vi "Generate All Combinations of N-Dimensional Coordinates Ver05.vi"(4 "Delete ROWS w/\nCOL #2 > #1":bool, 5 "Delete ROWS w/\nCOL #1 > #0":bool, 6 "INDEX of \nCOLS to Use":dbl[](array[numeric])=[0.0, 1.0, 2.0], 7 "Delete ROWS w/\nCOL #2 < #0":bool, 8 "Delete ROW if\nContains #":dbl=99.99, 10 "2D Big Data Array":dbl[][](array[numeric])=[[66.0, 11.0, 111.0], [2.0, 22.0, 9.0]]) -> (3 "FINAL ARRAY":dbl[][](array[numeric]))   [LabVIEW 2017]
uses:
  <vilib>/Analysis/Matrix/Numeric/Conversions/Array To Matrix - RA2.vi
  <vilib>/Analysis/Matrix/Numeric/Conversions/Matrix To Array - RM.vi
  <vilib>/Analysis/Matrix/NI_Matrix.lvlib
panel:
  in  "Tab Control":T1(tab)
  out "All COMBINATIONS of Numbers in Selected COLS":dbl[][](array[numeric])
  out "1st Condition Applied (Remove \nColumns with COL#1 > COL#0)":dbl[][](array[numeric])
  out "2nd Condition Applied (Remove \nColumns with COL#2 > COL#1)":dbl[][](array[numeric])
  out "FINAL # of ROWS":i32
  out "Selected COLS":dbl[][](array[numeric])
  out "# Dimensions \nSelected":i32
  # "COL#0"
  # "COL#1"
  # "COL#2"
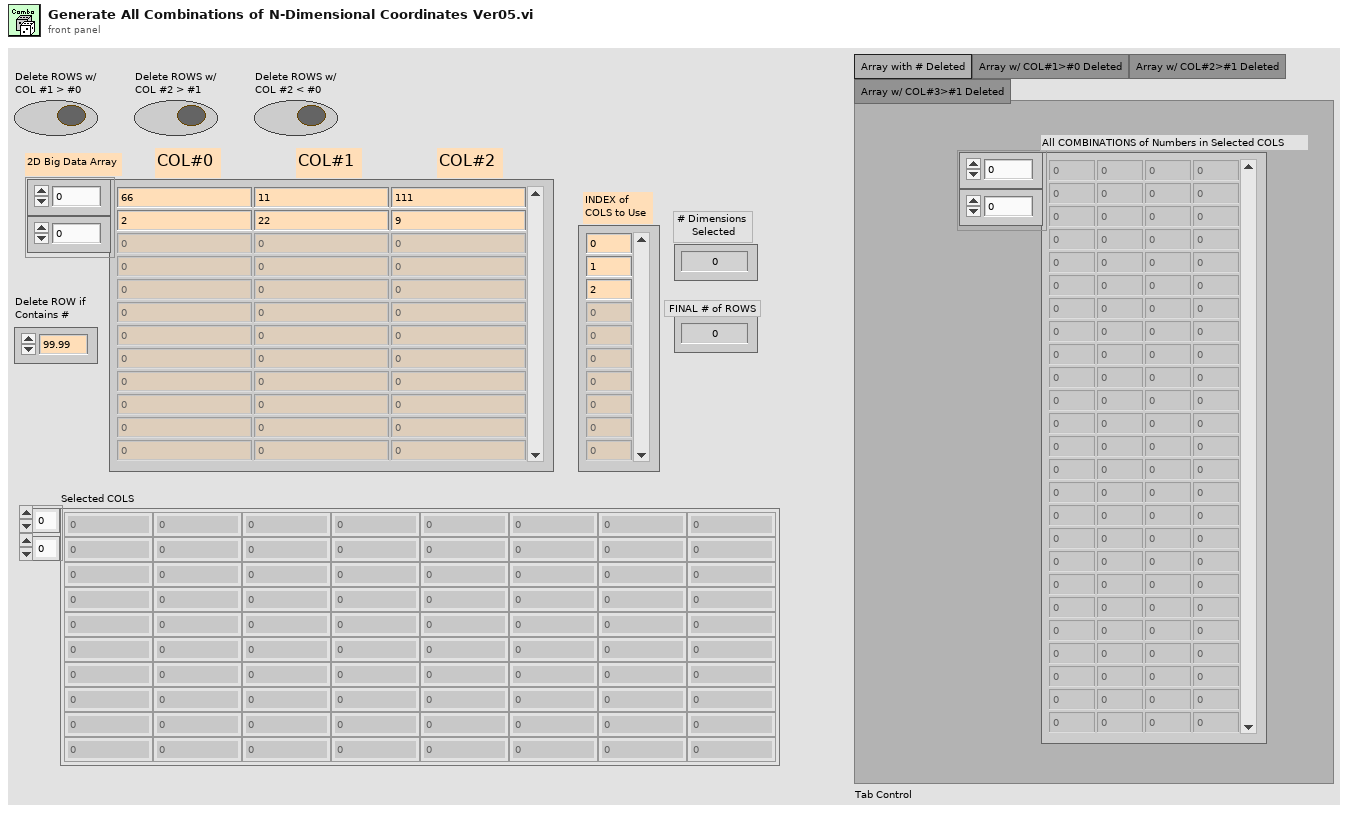
[diagram p1: front panel]
types:
  T1 = enum32{"Array with # Deleted", "Array w/ COL#1>#0 Deleted", "Array w/ COL#2>#1 Deleted", "Array w/ COL#3>#1 Deleted"}
  T2 = typedef "NI_Matrix.lvlib/RealMatrix.ctl" = dbl[][]
  T3 = cluster{"[0]":dbl, "[1]":dbl, "[2]":dbl, "[3]":dbl, "[4]":dbl, "[5]":dbl, "[6]":dbl, "[7]":dbl, "[8]":dbl}
  T4 = cluster{"[0]":dbl, "[1]":dbl, "[2]":dbl, "[3]":dbl, "[4]":dbl, "[5]":dbl, "[6]":dbl, "[7]":dbl, "[8]":dbl}[]
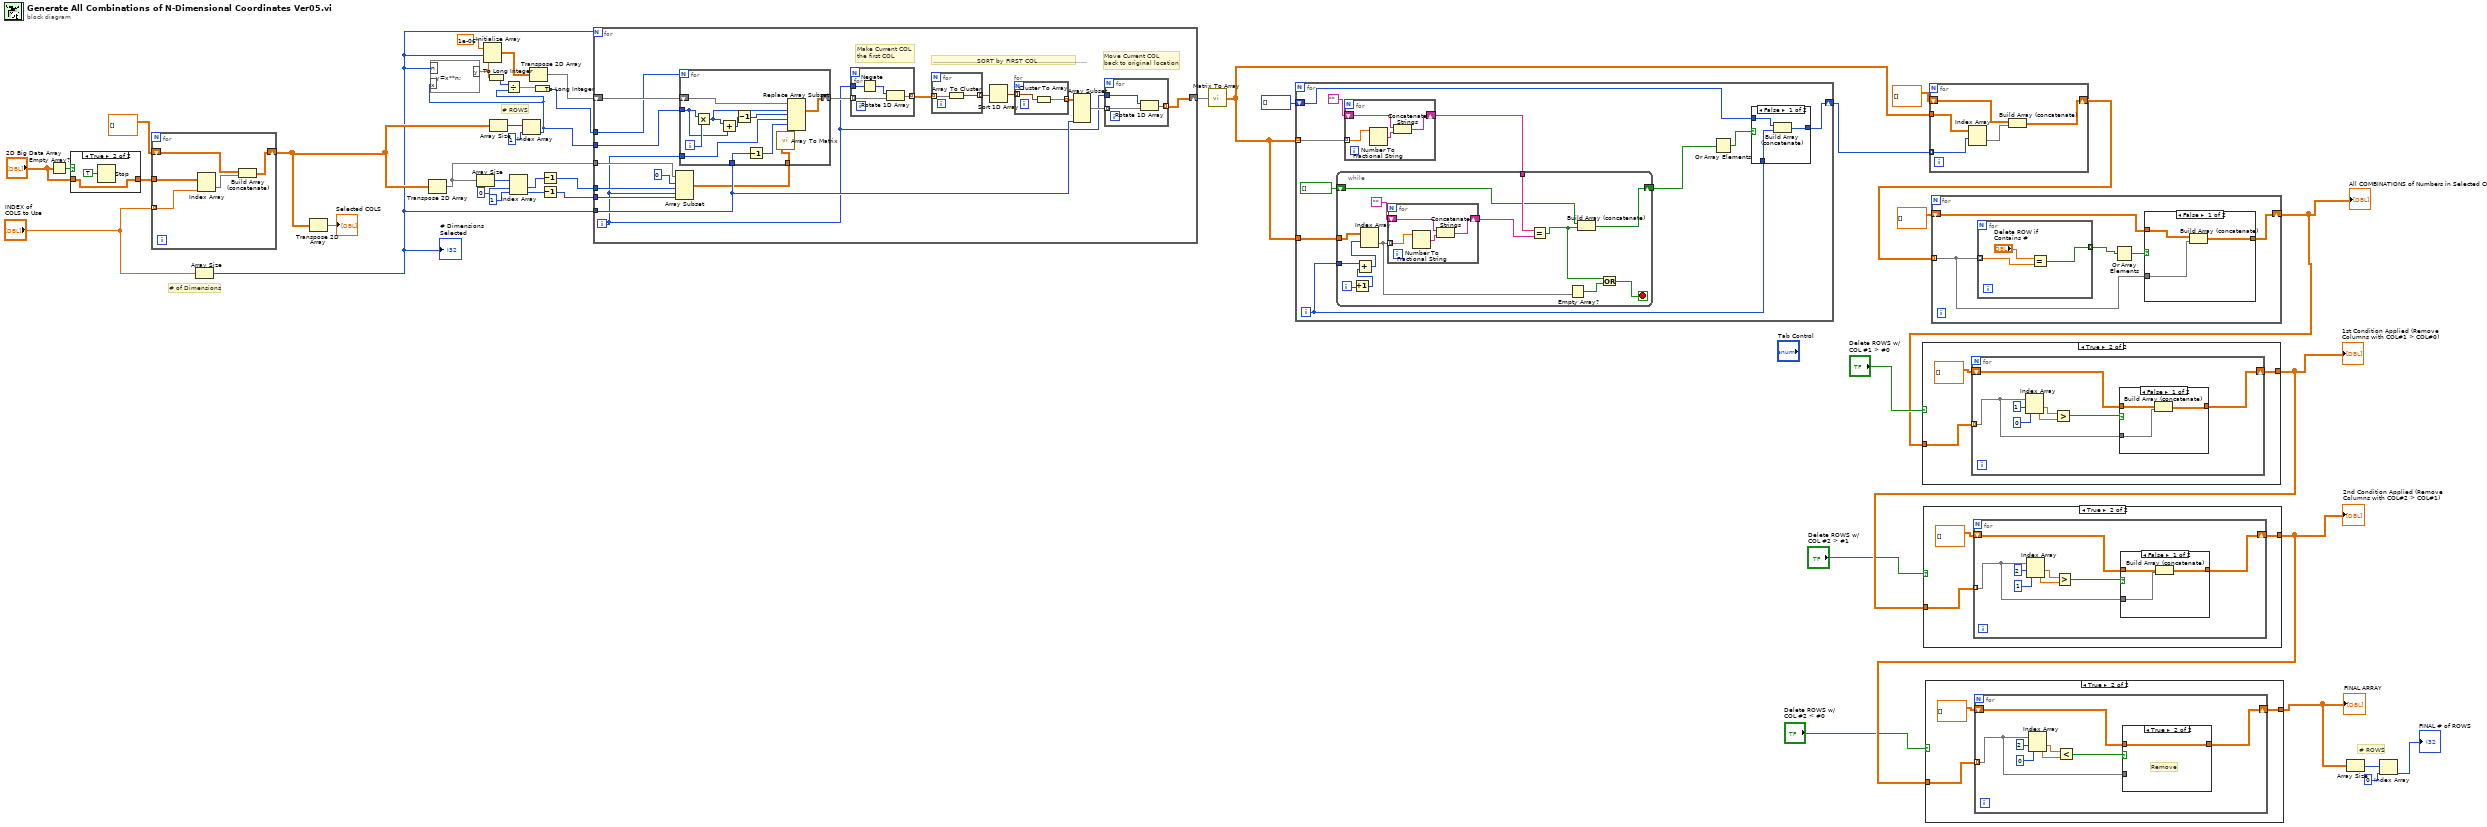
[diagram p0: block diagram]
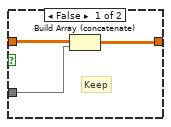
[diagram p3: hidden frame]
diagram:
  # "# ROWS"
  # "# ROWS"
  # "# of Dimensions"
  n1 = Empty Array?(array="2D Big Data Array") -> (empty?=w18:bool)
  n2 = case shown="True" w18 {
    tunnel: "2D Big Data Array" -> [w44 w45]
    tunnel: [w44 w45] -> w17
    frame False {
    }
    frame True {
      n3 = Stop(stop? (T)=TRUE) -> ()
    }
  }
  n4 = for {
    tunnel: w17 -> [w51]
    tunnel: "INDEX of \nCOLS to Use" -> [w50] mode=indexing
    shift-right: [w48] -> w34
    shift-left: dbl[][] [] -> [w47]
    n5 = Index Array(array=w51, index (col)=w50) -> (element=w49:dbl[])  [unwired: 1 in]
    n6 = Build Array (concatenate)(w47, w49) -> (w48:dbl[][])
  }
  n7 = Array Size(array="INDEX of \nCOLS to Use") -> (size(s)=w20:i32)
  "# Dimensions \nSelected" <- w20
  n8 = Transpose 2D Array(2D array=w34) -> (transposed array=→"Selected COLS":dbl[][])
  n9 = Transpose 2D Array(2D array=w34) -> (transposed array=w24:dbl[][])
  n10 = Array Size(array=w24) -> (size(s)=w28:i32[])
  n11 = Array Size(array=w34) -> (size(s)=w40:i32[])
  n12 = Index Array(array=w28, index #1=0 ("index"), index #2=1 ("index")) -> (element #1=w23:i32, element #2=w25:i32)
  n13 = Index Array(array=w40, index=1) -> (element=w29:i32)
  n14 = formula code="y=x**n;"("x"=w29, "n"=w20) -> ("y"=w33:dbl)
  n15 = Initialize Array(1e-06 ("element"), w20, w33) -> (w36:dbl[][])
  n16 = To Long Integer(number=w33) -> (32bit integer=w32:i32)
  n17 = Divide(x=w32, y=w29) -> (x/y=w31:dbl)
  n18 = Transpose 2D Array(2D array=w36) -> (transposed array=w35:dbl[][])
  n19 = To Long Integer(number=w31) -> (32bit integer=w30:i32)
  n20 = Decrement(x=w23) -> (x-1=w22:i32)
  n21 = Decrement(x=w25) -> (x-1=w21:i32)
  n22 = for {
    N: w20 -> [_]
    shift-right: [w52] -> w37
    shift-left: w35 -> [w64]
    tunnel: w30 -> [w61]
    tunnel: w20 -> [w65]
    tunnel: w29 -> [w62]
    tunnel: w24 -> [w59]
    tunnel: w22 -> [w58]
    tunnel: w21 -> [w57]
    i -> [w53]
    # "Move Current COL \nback to original location"
    # "......................SORT by FIRST COL........................."
    # "Make Current COL\nthe first COL"
    n23 = Array Subset(array=w59, index (row)=0 ("row 1"), length (row)=w58, index (col)=w53, length (col)=w57) -> (w63:dbl[][])
    n24 = for {
      N: w61 -> [_]
      tunnel: w62 -> [w84]
      shift-right: [w89] -> w56
      shift-left: w64 -> [w91]
      tunnel: w65 -> [w82]
      tunnel: w63 -> [w83]
      tunnel: w53 -> [w80]
      i -> [w90]
      n25 = Multiply(x=w84, y=w90) -> (x*y=w87:i32)
      n26 = Add(x=w87, y=w84) -> (x+y=w86:i32)
      n27 = Decrement(x=w86) -> (x-1=w85:i32)
      n28 = Decrement(x=w82) -> (x-1=w81:i32)
      n29 = call-poly <vilib>:"Array To Matrix.vi"("Real 2D Array"=w83) -> ("Real Matrix"=w88:T2)
      n30 = Replace Array Subset(array=w91, new element=w88, index (dim 0)=w87, index (dim 1)=w85, index (dim 2)=w80, index (dim 3)=w81) -> (w89:T2)
    }
    n31 = for {
      tunnel: w56 -> [w75] mode=indexing
      tunnel: w53 -> [w73]
      tunnel: [w74] -> w55 mode=indexing
      n32 = Negate(x=w73) -> (-x=w72:i32)
      n33 = Rotate 1D Array(1:w75, 2:w72) -> (0:w74:dbl[])
    }
    n34 = for {
      tunnel: w55 -> [w79] mode=indexing
      tunnel: [w78] -> w68 mode=indexing
      n35 = Array To Cluster(array=w79) -> (cluster=w78:T3)
    }
    n36 = Sort 1D Array(array=w68) -> (sorted array=w67:T4)
    n37 = for {
      tunnel: w67 -> [w77] mode=indexing
      tunnel: [w76] -> w66 mode=indexing
      n38 = Cluster To Array(cluster=w77) -> (array=w76:dbl[])
    }
    n39 = Array Subset(array=w66, length (col)=w65) -> (w54:dbl[][])  [unwired: 3 in]
    n40 = for {
      tunnel: w54 -> [w71] mode=indexing
      tunnel: [w70] -> w52 mode=indexing
      tunnel: w53 -> [w69]
      n41 = Rotate 1D Array(1:w71, 2:w69) -> (0:w70:dbl[])
    }
  }
  n42 = call-poly <vilib>:"Matrix To Array.vi"("Real Matrix"=w37) -> ("Real 2D Array"=w15:dbl[][])
  n43 = for {
    tunnel: w15 -> [w101] mode=indexing
    shift-right: [w94] -> w14
    shift-left: i32[] [] -> [w93]
    tunnel: w15 -> [w99]
    i -> [w95]
    n44 = for {
      tunnel: w101 -> [w127] mode=indexing
      shift-right: [w124] -> w98
      shift-left: "" -> [w125]
      n45 = Number To Fractional String(number=w127) -> (F-format string=w126:string)  [unwired: 3 in]
      n46 = Concatenate Strings(w125, w126) -> (w124:string)
    }
    n47 = while {
      tunnel: w99 -> [w118]
      tunnel: w98 -> [w117]
      tunnel: w95 -> [w115]
      shift-right: [w111] -> w96
      shift-left: bool[] [] -> [w112]
      i -> [w107]
      stop <- w108 stop-if-true
      n48 = Increment(x=w107) -> (x+1=w106:i32)
      n49 = Add(x=w115, y=w106) -> (x+y=w114:i32)
      n50 = Index Array(array=w118, index (row)=w114) -> (element=w113:dbl[])  [unwired: 1 in]
      n51 = for {
        tunnel: w113 -> [w123] mode=indexing
        shift-right: [w120] -> w116
        shift-left: "" -> [w121]
        n52 = Number To Fractional String(number=w123) -> (F-format string=w122:string)  [unwired: 3 in]
        n53 = Concatenate Strings(w121, w122) -> (w120:string)
      }
      n54 = Equal?(x=w117, y=w116) -> (x = y?=w109:bool)
      n55 = Empty Array?(array=w113) -> (empty?=w110:bool)
      n56 = Build Array (concatenate)(w112, w109) -> (w111:bool[])
      n57 = Or(x=w109, y=w110) -> (x .or. y?=w108:bool)
    }
    n58 = Or Array Elements(Boolean array=w96) -> (logical OR=w92:bool)
    n59 = case shown="False" w92 {
      tunnel: w95 -> [w104 _]
      tunnel: [w103 w105] -> w94
      tunnel: w93 -> [w102 w105]
      frame False {
        n60 = Build Array (concatenate)(w102, w104) -> (w103:i32[])
      }
      frame True {
      }
    }
  }
  n61 = for {
    tunnel: w15 -> [w131]
    shift-right: [w129] -> w9
    shift-left: dbl[][] [] -> [w128]
    tunnel: w14 -> [w132] mode=indexing
    n62 = Index Array(array=w131, index (row)=w132) -> (element=w130:dbl[])  [unwired: 1 in]
    n63 = Build Array (concatenate)(w128, w130) -> (w129:dbl[][])
  }
  n64 = for {
    tunnel: w9 -> [w135] mode=indexing
    shift-right: [w134] -> w6
    shift-left: dbl[][] [] -> [w133]
    n65 = for {
      tunnel: w135 -> [w144] mode=indexing
      tunnel: [w142] -> w137 mode=indexing
      n66 = Equal?(x="Delete ROW if\nContains #", y=w144) -> (x = y?=w142:bool)
    }
    n67 = Or Array Elements(Boolean array=w137) -> (logical OR=w136:bool)
    n68 = case shown="False" w136 {
      tunnel: w135 -> [w140 _]
      tunnel: [w139 w141] -> w134
      tunnel: w133 -> [w138 w141]
      frame False {
        n69 = Build Array (concatenate)(w138, w140) -> (w139:dbl[][])
      }
      frame True {
      }
    }
  }
  "All COMBINATIONS of Numbers in Selected COLS" <- w6
  n70 = case shown="True" "Delete ROWS w/\nCOL #1 > #0" {
    tunnel: w6 -> [w145 w147]
    tunnel: [w145 w146] -> w5
    frame False {
    }
    frame True {
      n71 = for {
        shift-right: [w151] -> w146
        shift-left: dbl[][] [] -> [w150]
        tunnel: w147 -> [w149] mode=indexing
        n72 = Index Array(array=w149, index #1=1 ("index"), index #2=0 ("index")) -> (element #1=w154:dbl, element #2=w153:dbl)
        n73 = Greater?(x=w154, y=w153) -> (0:w152:bool)
        n74 = case shown="False" w152 {
          tunnel: [w157 w160] -> w151
          tunnel: w150 -> [w159 w160]
          tunnel: w149 -> [w158 _]
          frame False {
            n75 = Build Array (concatenate)(w159, w158) -> (w157:dbl[][])
          }
          frame True {
          }
        }
      }
    }
  }
  "1st Condition Applied (Remove \nColumns with COL#1 > COL#0)" <- w5
  n76 = case shown="True" "Delete ROWS w/\nCOL #2 > #1" {
    tunnel: w5 -> [w161 w163]
    tunnel: [w161 w162] -> w3
    frame False {
    }
    frame True {
      n77 = for {
        shift-right: [w167] -> w162
        shift-left: dbl[][] [] -> [w166]
        tunnel: w163 -> [w165] mode=indexing
        n78 = Index Array(array=w165, index #1=2 ("index"), index #2=1 ("index")) -> (element #1=w170:dbl, element #2=w169:dbl)
        n79 = Greater?(x=w170, y=w169) -> (0:w168:bool)
        n80 = case shown="False" w168 {
          tunnel: [w173 w176] -> w167
          tunnel: w166 -> [w175 w176]
          tunnel: w165 -> [w174 _]
          frame False {
            n81 = Build Array (concatenate)(w175, w174) -> (w173:dbl[][])
          }
          frame True {
          }
        }
      }
    }
  }
  "2nd Condition Applied (Remove \nColumns with COL#2 > COL#1)" <- w3
  n82 = case shown="True" "Delete ROWS w/\nCOL #2 < #0" {
    tunnel: w3 -> [w177 w179]
    tunnel: [w177 w178] -> w1
    frame False {
    }
    frame True {
      n83 = for {
        shift-right: [w183] -> w178
        shift-left: dbl[][] [] -> [w182]
        tunnel: w179 -> [w181] mode=indexing
        n84 = Index Array(array=w181, index #1=2 ("index"), index #2=0 ("index")) -> (element #1=w186:dbl, element #2=w185:dbl)
        n85 = Less?(x=w186, y=w185) -> (x < y?=w184:bool)
        n86 = case shown="True" w184 {
          tunnel: [w189 w192] -> w183
          tunnel: w182 -> [w191 w192]
          tunnel: w181 -> [w190 _]
          frame False {
            # "Keep"
            n87 = Build Array (concatenate)(w191, w190) -> (w189:dbl[][])
          }
          frame True {
            # "Remove"
          }
        }
      }
    }
  }
  "FINAL ARRAY" <- w1
  n88 = Array Size(array=w1) -> (size(s)=w12:i32[])
  n89 = Index Array(array=w12, index=0) -> (element=→"FINAL # of ROWS":i32)
